vi "RSZVB Set Discrete Marker.vi"(7 "Discrete Mode (0: Continuous)":i32(ring) items=["Continuous", "Discrete"], 8 "error in (no error)":errorcluster {"code" format="%.0x"}, 9 "Marker (1)":i32=1, 10 "Channel (Trace) (1)":i32=1, 11 "VISA session":refnum<visa-resource-name>) -> (0 "error out":errorcluster {"code" format="%.0x"}, 3 "dup VISA session":refnum<visa-resource-name>)   [LabVIEW 2011]
doc: "This VI sets marker no. <Mk> to continuous or discrete mode. The marker doesn't have to be created before (CALCulate<Ch/Tr>:MARKer<Mk>[:STATe] ON), the mode can be assigned in advance.\n\nRemote-control command(s):\nCALCulate<Ch/Tr>:MARKer<Mk>:MODE CONTinuous | DISCrete"
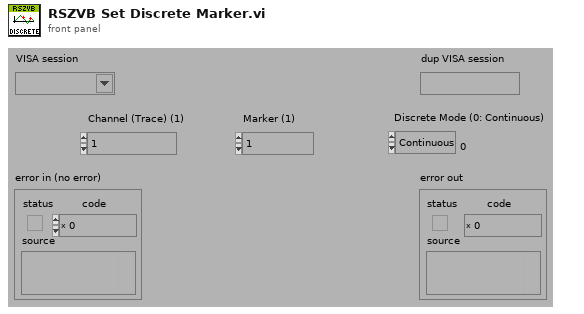
[diagram p1: front panel]
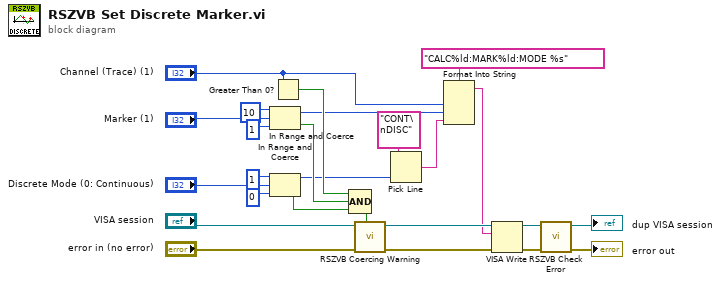
[diagram p0: block diagram]
diagram:
  n1 = In Range and Coerce(upper limit=10, x="Marker (1)", lower limit=1) -> (coerced(x)=w14:i32, In Range?=w15:bool)
  n2 = In Range and Coerce(upper limit=1, x="Discrete Mode (0: Continuous)", lower limit=0) -> (coerced(x)=w2:i32, In Range?=w4:bool)
  n3 = Greater Than 0?(x="Channel (Trace) (1)") -> (x > 0?=w18:bool)
  n4 = Compound Arithmetic op=AND(w18, w15, w4) -> (w20:bool)
  n5 = call "RSZVB Coercing Warning.vi"("In Range?"=w20, "error in (no error)"="error in (no error)", "VISA session"="VISA session") -> ("error out"=w23:errorcluster, "dup VISA session"=w24:refnum<visa-resource-name>)  [unwired: 7 in]
  n6 = Pick Line(multi-line string="CONT\nDISC", line index=w2) -> (output string=w1:string)  [unwired: 1 in]
  n7 = Format Into String(format string="CALC%ld:MARK%ld:MODE %s", "Channel (Trace) (1)", w14, w1) -> (resulting string=w19:string)  [unwired: 2 in, 1 out]
  n8 = VISA Write(VISA resource name=w24, write buffer=w19, error in (no error)=w23) -> (VISA resource name out=w21:refnum<visa-resource-name>, error out=w22:errorcluster)  [unwired: 1 out]
  n9 = call "RSZVB Check Error.vi"("error in (no error)"=w22, "VISA session"=w21) -> ("error out"=→"error out":errorcluster, "dup VISA session"=→"dup VISA session":refnum<visa-resource-name>)  [unwired: 8 in]
